vi "toString.vi"(8 "error in (no error)":errorcluster, 11 "Record in":refnum<class "Record.lvclass">) -> (0 "error out":errorcluster, 2 "String":string, 3 "Record out":refnum<class "Record.lvclass">)   [LabVIEW 2017, in "Error Log.lvlib" / "Record.lvclass"]
uses:
  Record.lvclass
  Record.lvclass/Record.ctl
  Serializer/Serializer.lvclass
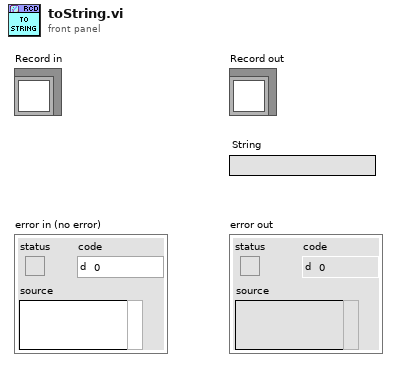
[diagram p1: front panel]
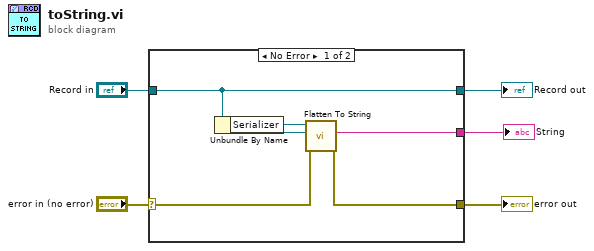
[diagram p0: block diagram]
diagram:
  n1 = case shown="No Error" "error in (no error)" {
    selector: "error in (no error)" -> [w7 w12]
    tunnel: [w6 w12] -> w4
    tunnel: [w9 w11] -> w1
    tunnel: "Record in" -> [w9 w11]
    tunnel: [w8 _] -> w2
    frame No Error {
      n2 = Unbundle By Name(w9) -> ("Serializer"=w10:refnum<class "Serializer.lvclass">)
      n3 = call "Flatten To String.vi"("error in (no error)"=w7, "Record"=w9, "Serializer in"=w10) -> ("error out"=w6:errorcluster, "Flattened String"=w8:string)  [unwired: 6 in, 1 out]
    }
    frame Error {
    }
  }
  "error out" <- w4
  "Record out" <- w1
  "String" <- w2
